vi "TSCAN_CAN_Fold.vi"(10 "Buffer":T1(array[cluster]), 11 "Fold Data":bool) -> (2 "Buffer out":T1(array[cluster]))   [LabVIEW 2014]
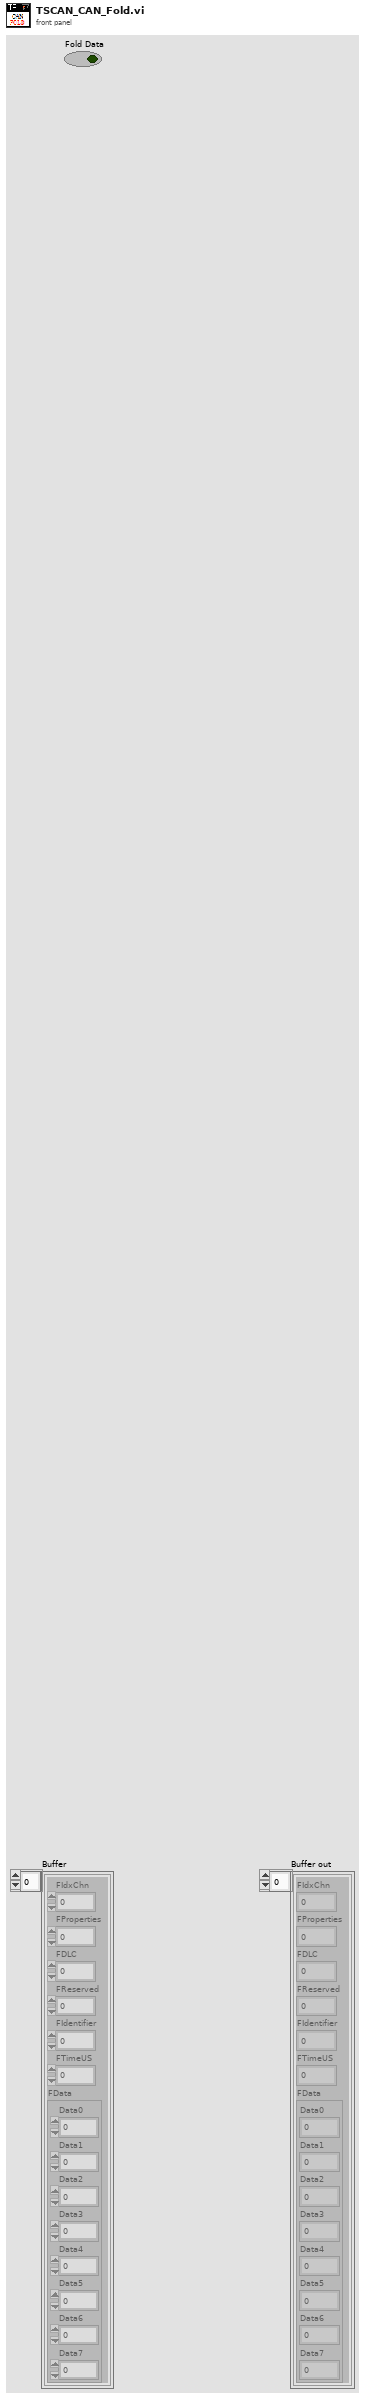
[diagram p1: front panel]
types:
  T1 = cluster{"FIdxChn":u8, "FProperties":u8, "FDLC":u8, "FReserved":u8, "FIdentifier":i32, "FTimeUS":u64, "FData":cluster{"Data0":u8, "Data1":u8, "Data2":u8, "Data3":u8, "Data4":u8, "Data5":u8, "Data6":u8, "Data7":u8}}[]
  T2 = cluster{"FIdxChn":u8, "FProperties":u8, "FDLC":u8, "FReserved":u8, "FIdentifier":i32, "FTimeUS":u64, "FData":cluster{"Data0":u8, "Data1":u8, "Data2":u8, "Data3":u8, "Data4":u8, "Data5":u8, "Data6":u8, "Data7":u8}}
  T3 = cluster{"FDLC":u8, "簇":cluster{"FIdxChn":u8, "FProperties":u8, "FDLC":u8, "FReserved":u8, "FIdentifier":i32, "FTimeUS":u64, "FData":cluster{"Data0":u8, "Data1":u8, "Data2":u8, "Data3":u8, "Data4":u8, "Data5":u8, "Data6":u8, "Data7":u8}}}
  T4 = cluster{"FDLC":u8, "簇":cluster{"FIdxChn":u8, "FProperties":u8, "FDLC":u8, "FReserved":u8, "FIdentifier":i32, "FTimeUS":u64, "FData":cluster{"Data0":u8, "Data1":u8, "Data2":u8, "Data3":u8, "Data4":u8, "Data5":u8, "Data6":u8, "Data7":u8}}}[]
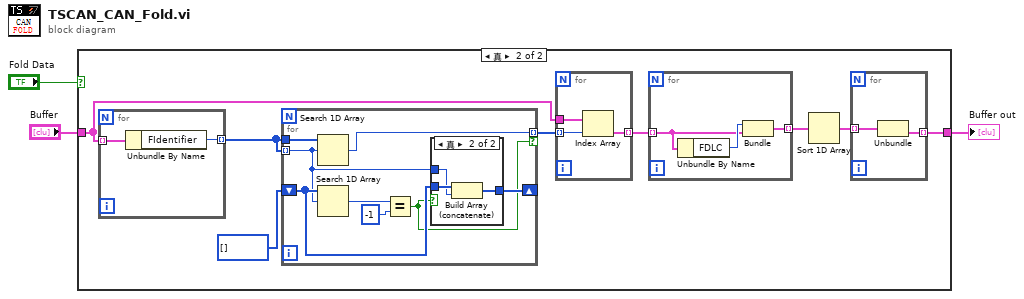
[diagram p0: block diagram]
diagram:
  n1 = case shown="真" "Fold Data" {
    tunnel: [w4 w11] -> w1
    tunnel: "Buffer" -> [w4 w5]
    frame False {
    }
    frame True {
      n2 = for {
        tunnel: w5 -> [w29] mode=indexing
        tunnel: [w28] -> w8 mode=indexing
        n3 = Unbundle By Name(w29) -> ("FIdentifier"=w28:i32)
      }
      n4 = for {
        tunnel: w8 -> [w18] mode=indexing
        shift-right: [w23] -> _
        shift-left: u32[] [] -> [w22]
        tunnel: [w17] -> w6 mode=indexing if=w16
        tunnel: w8 -> [w19]
        n5 = Search 1D Array(1D array=w19, element=w18) -> (index of element=w17:i32)  [unwired: 1 in]
        n6 = Search 1D Array(1D array=w22, element=w18) -> (index of element=w20:i32)  [unwired: 1 in]
        n7 = Equal?(x=w20, y=-1) -> (x = y?=w16:bool)
        n8 = case shown="真" w16 {
          tunnel: [w24 w25] -> w23
          tunnel: w22 -> [w24 w27]
          tunnel: w18 -> [_ w26]
          frame False {
          }
          frame True {
            n9 = Build Array (concatenate)(w27, w26) -> (w25:u32[])
          }
        }
      }
      n10 = for {
        tunnel: w5 -> [w15]
        tunnel: w6 -> [w14] mode=indexing
        tunnel: [w13] -> w12 mode=indexing
        n11 = Index Array(array=w15, index=w14) -> (element=w13:T2)
      }
      n12 = for {
        tunnel: w12 -> [w33] mode=indexing
        tunnel: [w32] -> w10 mode=indexing
        n13 = Unbundle By Name(w33) -> ("FDLC"=w34:u8)
        n14 = Bundle("FDLC"=w34, "簇"=w33) -> (w32:T3)  [unwired: 1 in]
      }
      n15 = Sort 1D Array(array=w10) -> (sorted array=w9:T4)
      n16 = for {
        tunnel: w9 -> [w31] mode=indexing
        tunnel: [w30] -> w11 mode=indexing
        n17 = Unbundle(w31) -> ("簇"=w30:T2)  [unwired: 1 out]
      }
    }
  }
  "Buffer out" <- w1
